vi "test.vi"() -> ()   [LabVIEW 2016]
panel:
  out "Array 3":dbl[][](array[numeric])
  out "Array 2":dbl[][](array[numeric])
  in  "Weight Matrix #":i32
  out "Array":dbl[][](array[numeric])
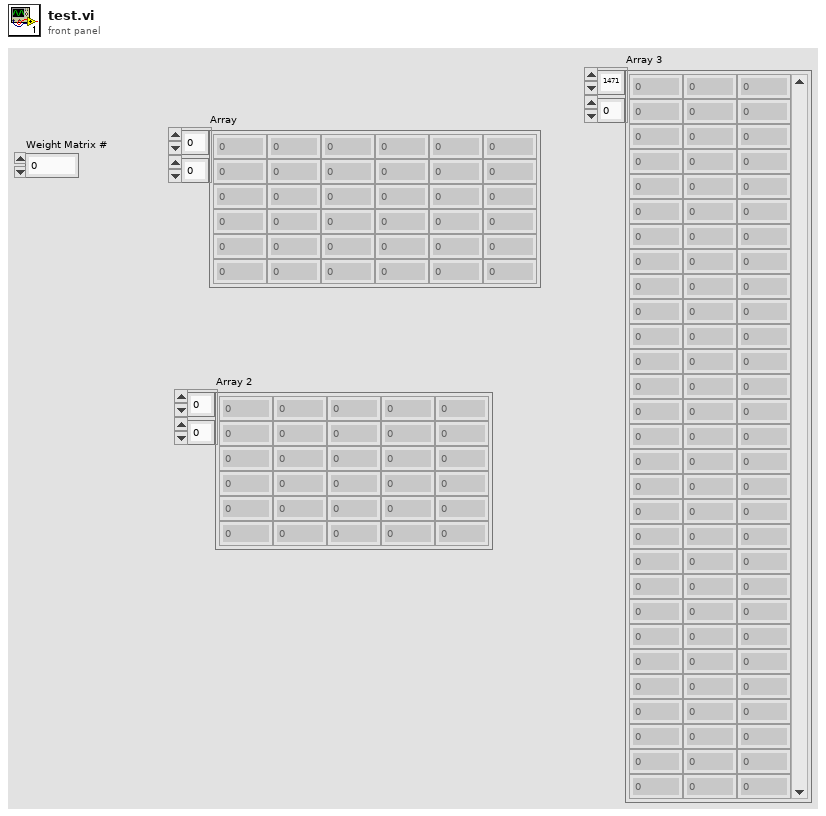
[diagram p1: front panel]
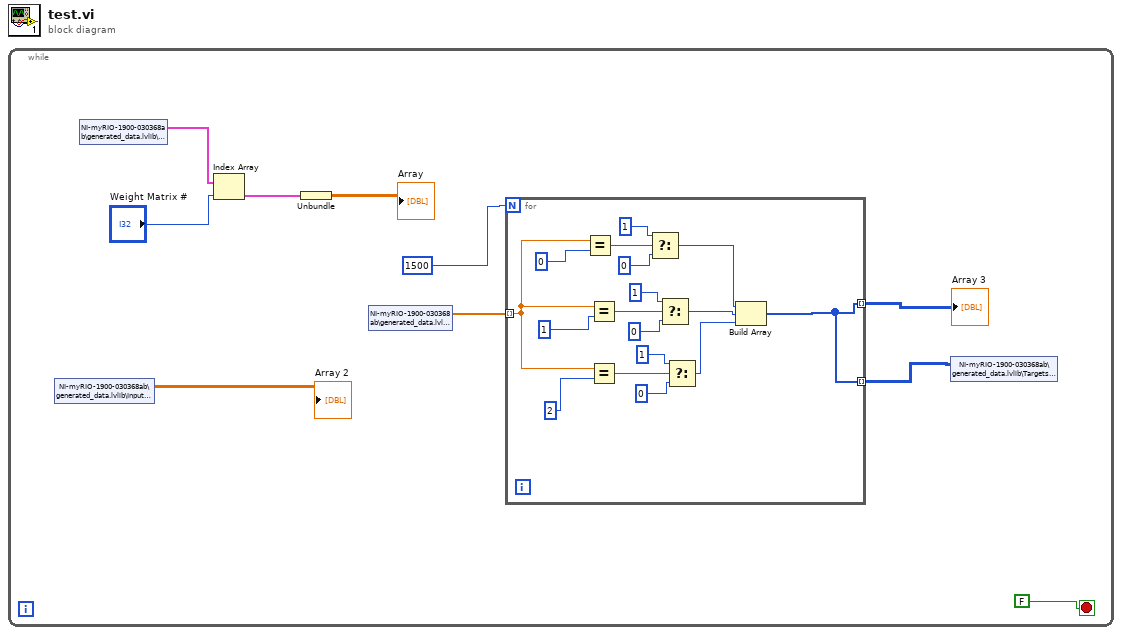
[diagram p0: block diagram]
diagram:
  n1 = while {
    stop <- FALSE stop-if-true
    n2 = shared-variable "NI-myRIO-1900-030368ab\\generated_data.lvlib\\Input Data"() -> (→"Array 2":dbl[][])  [unwired: 1 in, 1 out]
    n3 = shared-variable "NI-myRIO-1900-030368ab\\generated_data.lvlib\\Weights"() -> (w10:cluster{dbl[][]}[])  [unwired: 1 in, 1 out]
    n4 = Index Array(array=w10, index="Weight Matrix #") -> (element=w7:cluster{dbl[][]})
    n5 = Unbundle(w7) -> (→"Array":dbl[][])
    n6 = shared-variable "NI-myRIO-1900-030368ab\\generated_data.lvlib\\Targets"() -> (w4:dbl[])  [unwired: 1 in, 1 out]
    n7 = for {
      N: 1500 -> [_]
      tunnel: w4 -> [w26] mode=indexing
      tunnel: [w11] -> w2 mode=indexing
      tunnel: [w11] -> w1 mode=indexing
      n8 = Equal?(x=w26, y=0) -> (x = y?=w23:bool)
      n9 = Equal?(x=w26, y=1) -> (x = y?=w15:bool)
      n10 = Equal?(x=w26, y=2) -> (x = y?=w16:bool)
      n11 = Select(t=1, s=w23, f=0) -> (s? t:f=w14:i32)
      n12 = Select(t=1, s=w15, f=0) -> (s? t:f=w13:i32)
      n13 = Select(t=1, s=w16, f=0) -> (s? t:f=w12:i32)
      n14 = Build Array(w14, w13, w12) -> (w11:i32[])
    }
    "Array 3" <- w2
    n15 = shared-variable "NI-myRIO-1900-030368ab\\generated_data.lvlib\\Targets_OH"(w1) -> ()  [unwired: 1 in, 1 out]
  }
